vi "Read Bytes Until Buffer Empty.vi"(8 "error in":errorcluster, 10 "timeout (ms)":i32=-1, 11 "MC VISA resource in":refnum<visa-resource-name>) -> (0 "error out":errorcluster, 2 "read buffer":string, 3 "MC VISA resource  out":refnum<visa-resource-name>)   [LabVIEW 2009]
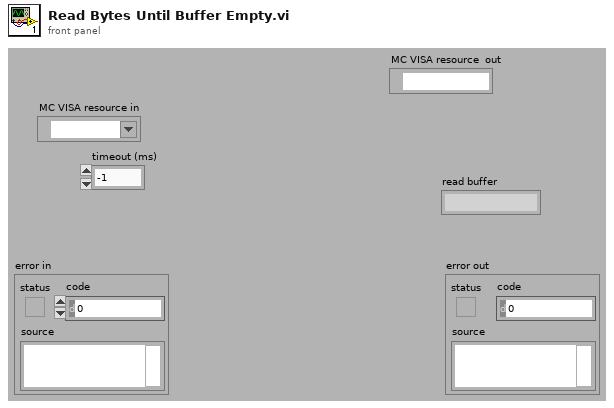
[diagram p1: front panel]
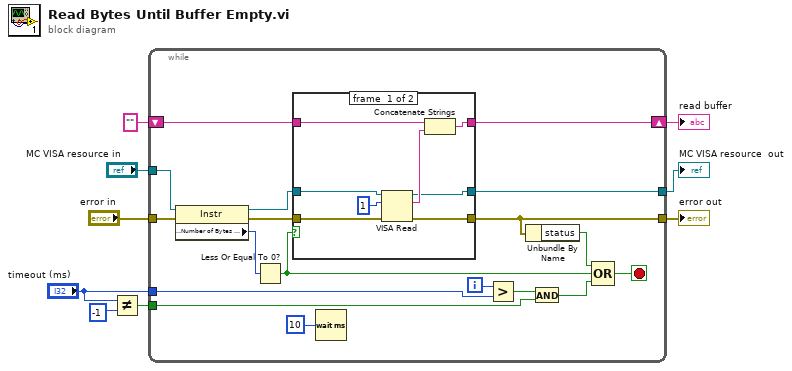
[diagram p0: block diagram]
diagram:
  n1 = Not Equal?(x="timeout (ms)", y=-1) -> (x != y?=w1:bool)
  n2 = while {
    shift-right: [w20] -> w4
    shift-left: "" ("write buffer") -> [w24]
    tunnel: [w19] -> w5
    tunnel: [w23] -> w6
    tunnel: "MC VISA resource in" -> [w22]
    tunnel: "error in" -> [w21]
    tunnel: "timeout (ms)" -> [w14]
    tunnel: w1 -> [w10]
    i -> [w15]
    stop <- w18 stop-if-true
    n3 = property class="Instr"(reference=w22, error in=w21) -> (reference out=w25:refnum<visa-resource-name>, error out=w26:errorcluster, "Serial Settings:Number of Bytes at Serial Port"=w27:u32)
    n4 = Less Or Equal To 0?(x=w27) -> (x <= 0?=w13:bool)
    n5 = case shown="False" w13 {
      tunnel: w26 -> [w35 w36]
      tunnel: w25 -> [w34 w37]
      tunnel: w24 -> [w32 w38]
      tunnel: [w31 w36] -> w19
      tunnel: [w30 w37] -> w23
      tunnel: [w29 w38] -> w20
      frame #0 {
        n6 = VISA Read(VISA resource name=w34, byte count=u32 1, error in (no error)=w35) -> (VISA resource name out=w30:refnum<visa-resource-name>, read buffer=w33:string, error out=w31:errorcluster)  [unwired: 1 out]
        n7 = Concatenate Strings(w32, w33) -> (w29:string)
      }
      frame #1 {
      }
    }
    n8 = Wait (ms)(milliseconds to wait=u32 10) -> ()  [unwired: 1 out]
    n9 = Greater?(x=w15, y=w14) -> (0:w12:bool)
    n10 = Unbundle By Name(w19) -> ("status"=w17:bool)
    n11 = And(x=w12, y=w10) -> (x .and. y?=w11:bool)
    n12 = Compound Arithmetic op=OR(w17, w13, w11) -> (w18:bool)
  }
  "error out" <- w5
  "MC VISA resource  out" <- w6
  "read buffer" <- w4
